vi "Main.vi"() -> ()   [LabVIEW 2013]
doc: "This template is for the Queued Message Handler design pattern.\n\nThe Event Handling Loop generates messages based on user interface actions.\n\nThe Message Handling Loop processes messages generated by the Event Handling Loop, or by other messages. The messages are string values, so new messages can be added easily to the Message Cases case structure in the Message Handling Loop. Each message cluster can also provide an optional value for Message Data, which is a variant that can be converted to whatever message-specific data is required."
uses:
  controls/UI Data.ctl
  support/Message Queue/Enqueue Message (Single).vi
  support/Message Queue/Enqueue Message (Array).vi
  <vilib>/Utility/error.llb/Error Cluster From Error Code.vi
  <vilib>/ErrorRing/Error Ring.xnode
  support/Message Queue/Message Queue.lvlib
  support/User Event - Stop/User Event - Stop.lvlib
panel:
  out "Praca":bool
  out "Display <Replace Me>":string
  in  "Do Something Else <Replace Me>":bool
  in  "Do Something <Replace Me>":bool
  in  "Exit":bool
  # "These controls have associated \"Value Changed\" events configured in the Event Structure on the diagram.\n\nReplace them (and reconfigure the Event Structure) with the controls you need for your application."
  # "This template is for the Queued Message Handler design pattern.\n\nSee the block diagram for more information on how to use this template."
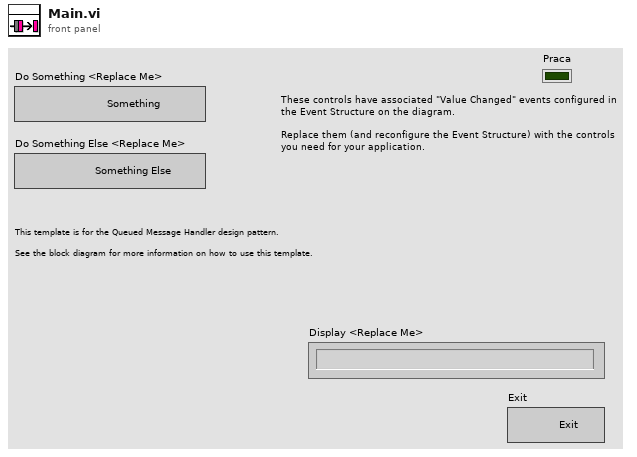
[diagram p1: front panel]
types:
  T1 = typedef "UI Data.ctl" = cluster{"Boolean <Replace Me>":bool, "String <Replace Me>":string, "Numeric <Replace Me>":dbl, "Do Something Ref":refnum<vi>, "Do Something Else Ref":refnum<vi>, "Data Display Ref":refnum<vi>, "Exit Button Ref":refnum<vi>}
  T2 = typedef "Message Queue.lvlib/All Message Queues.ctl" = cluster{"UI":refnum<queue>}
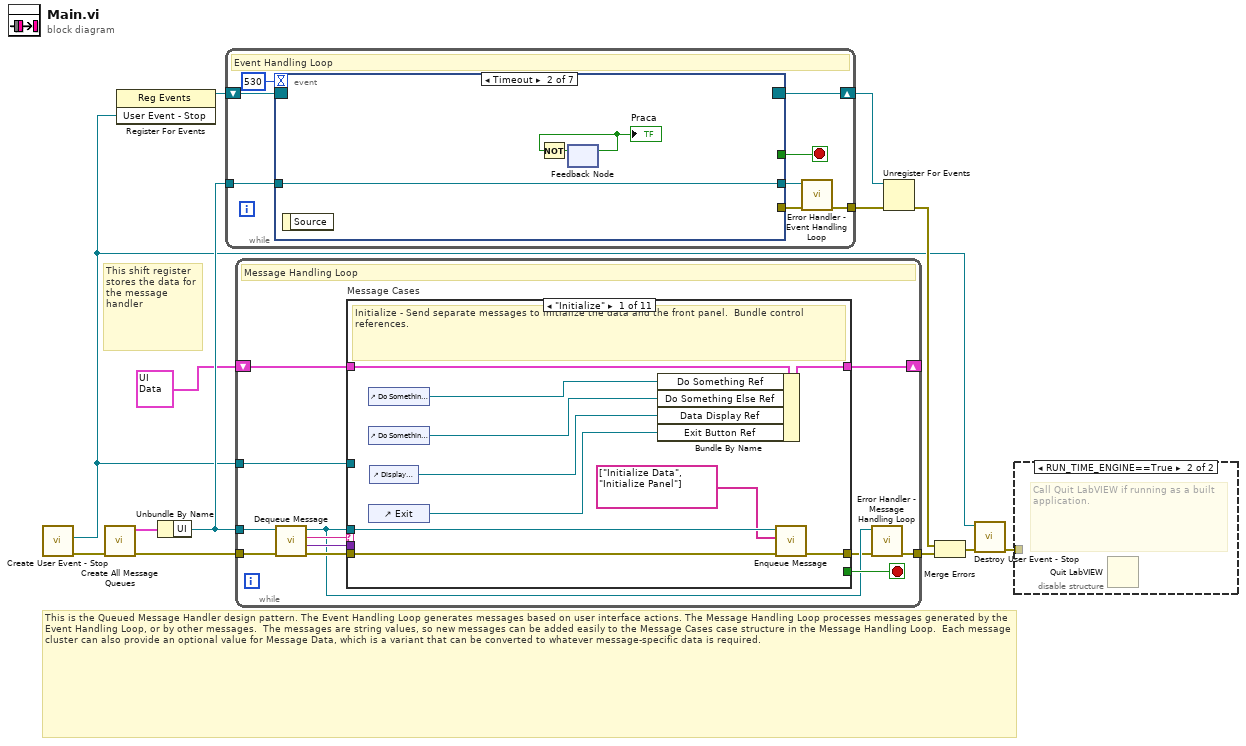
[diagram p0: block diagram]
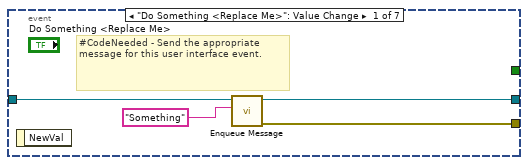
[diagram p3: hidden frame]
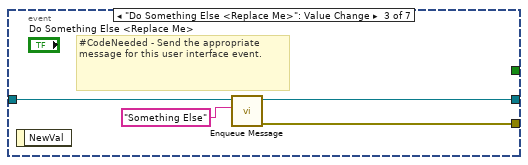
[diagram p4: hidden frame]
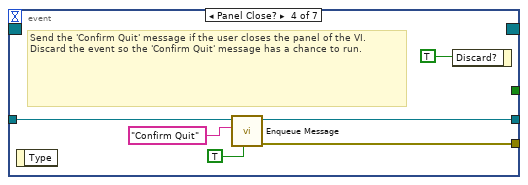
[diagram p5: hidden frame]
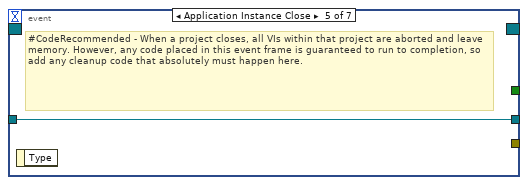
[diagram p6: hidden frame]
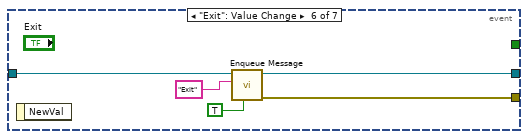
[diagram p7: hidden frame]
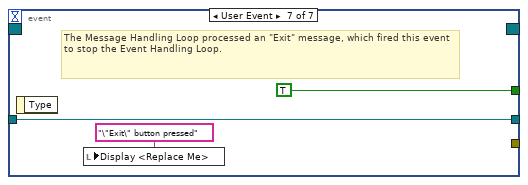
[diagram p8: hidden frame]
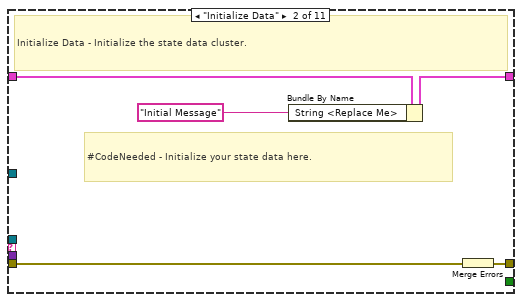
[diagram p9: hidden frame]
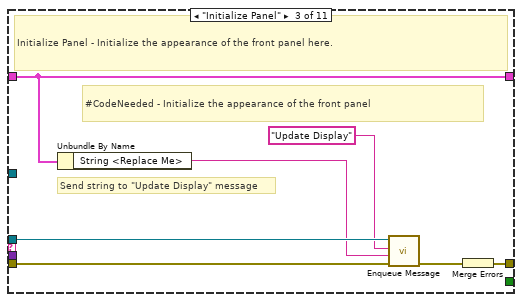
[diagram p10: hidden frame]
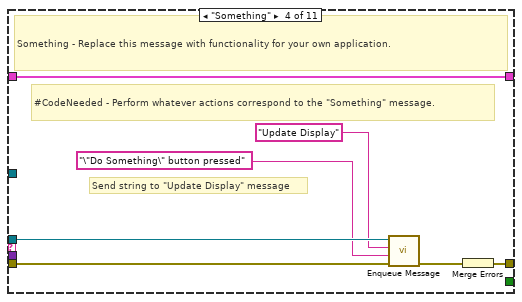
[diagram p11: hidden frame]
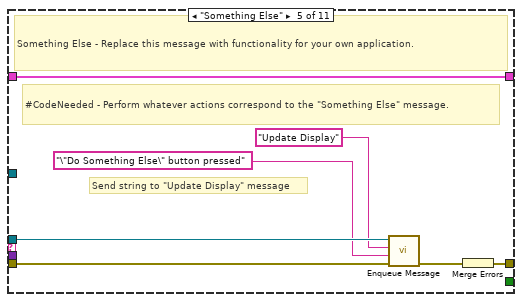
[diagram p12: hidden frame]
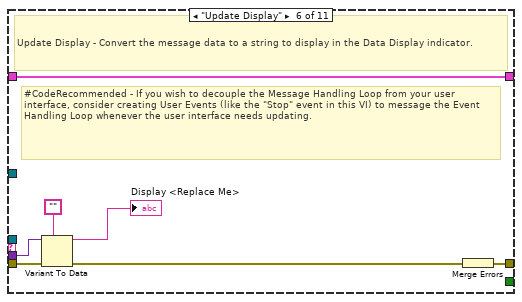
[diagram p13: hidden frame]
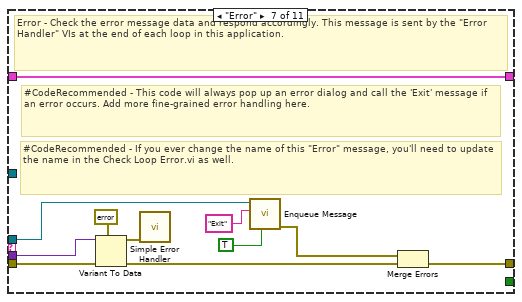
[diagram p14: hidden frame]
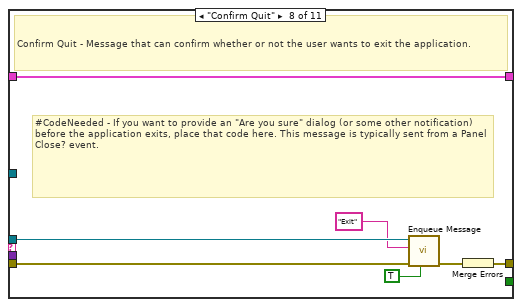
[diagram p15: hidden frame]
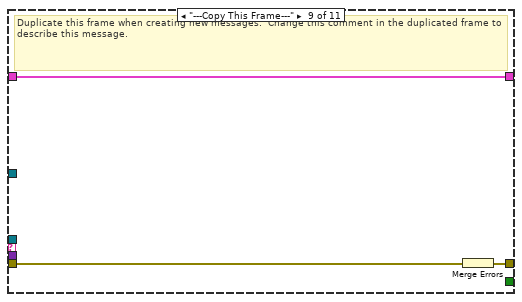
[diagram p16: hidden frame]
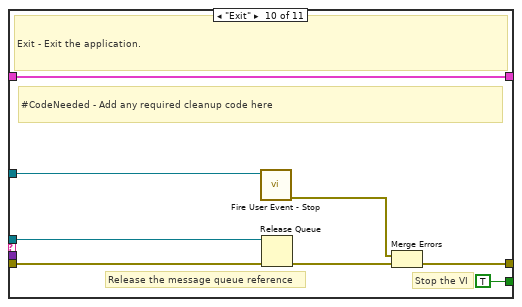
[diagram p17: hidden frame]
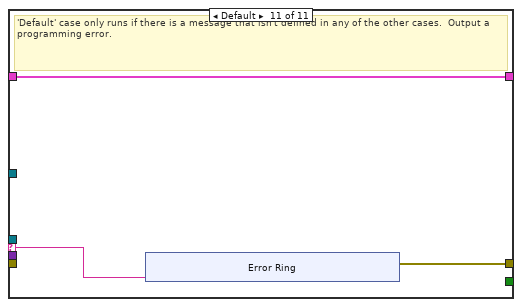
[diagram p18: hidden frame]
diagram:
  # "This is the Queued Message Handler design pattern. The Event Handling Loop generates messages based on user interface actions. The Message Handling Loop processes messages generated by the Event Handling Loop, or by other messages.  The messages are string values, so new messages can be added easily to the Message Cases case structure in the Message Handling Loop.  Each message cluster can also provide an optional value for Message Data, which is a variant that can be converted to whatever message-specific data is required."
  # "This shift register stores the data for the message handler"
  n1 = call "Create User Event - Stop.vi"() -> ("error out"=w9:errorcluster, "User Event - Stop"=w2:refnum<user-event>)  [unwired: 10 in]
  n2 = call "Create All Message Queues.vi"("error in (no error)"=w9) -> ("error out"=w13:errorcluster, "Message Queues out"=w12:T2)  [unwired: 9 in]
  n3 = register-events(w2) -> (reference out=w1:refnum<event-registration>)  [unwired: 2 in, 1 out]
  n4 = Unbundle By Name(w12) -> ("UI"=w10:refnum<queue>)
  n5 = while {
    tunnel: w10 -> [w21]
    shift-right: [w19] -> w6
    shift-left: w1 -> [w20]
    tunnel: [w15] -> w3
    stop <- w17 stop-if-true
    # "Event Handling Loop"
    n6 = event shown="[1] Timeout" {
      selector: w20 -> [_ _ _ _ _ _ _]
      dyn-events: [_ _ _ _ _ _ _] -> w19
      timeout: 530 -> [_ _ _ _ _ _ _]
      tunnel: [_ _ _ _ _ _ TRUE ("Discard?")] -> w17
      tunnel: w21 -> [w25 w28 w32 w37 w39 w44 w47]
      tunnel: [w22 _ w29 w36 _ w43 _] -> w18
      tunnel: [w24 w28 w31 w35 w39 w42 w47] -> w16
      event "Do Something <Replace Me>": Value Change {
        # "#CodeNeeded - Send the appropriate message for this user interface event."
        n7 = event-data() -> ()  [unwired: 1 in, 1 out]
        n8 = call-poly "Enqueue Message.vi"("Message"="Something", "Message Queue"=w25) -> ("error out"=w22:errorcluster, "dup Message Queue"=w24:refnum<queue>)  [unwired: 8 in]
      }
      event Timeout {
        n9 = event-data() -> ()  [unwired: 1 in, 1 out]
        n10 = feedback #1() -> (w26:bool)  [unwired: 1 in]
        "Praca" <- w26
        n11 = Not(x=w26) -> (.not. x?=w27:bool)
        n12 = feedback-in #1(w27) -> ()
      }
      event "Do Something Else <Replace Me>": Value Change {
        # "#CodeNeeded - Send the appropriate message for this user interface event."
        n13 = event-data() -> ()  [unwired: 1 in, 1 out]
        n14 = call-poly "Enqueue Message.vi"("Message"="Something Else", "Message Queue"=w32) -> ("error out"=w29:errorcluster, "dup Message Queue"=w31:refnum<queue>)  [unwired: 8 in]
      }
      event Panel Close? {
        # "Send the 'Confirm Quit' message if the user closes the panel of the VI. Discard the event so the 'Confirm Quit' message has a chance to run."
        n15 = event-data() -> ()  [unwired: 1 in, 1 out]
        n16 = call-poly "Enqueue Message.vi"("Priority Message? (F)"=TRUE, "Message"="Confirm Quit", "Message Queue"=w37) -> ("error out"=w36:errorcluster, "dup Message Queue"=w35:refnum<queue>)  [unwired: 7 in]
        n17 = event-data("Discard?"=TRUE) -> ()  [unwired: 1 in, 1 out]
      }
      event Application Instance Close {
        # "#CodeRecommended - When a project closes, all VIs within that project are aborted and leave memory. However, any code placed in this event frame is guaranteed to run to completion, so add any cleanup code that absolutely must happen here."
        n18 = event-data() -> ()  [unwired: 1 in, 1 out]
      }
      event "Exit": Value Change {
        n19 = event-data() -> ()  [unwired: 1 in, 1 out]
        n20 = call-poly "Enqueue Message.vi"("Priority Message? (F)"=TRUE, "Message"="Exit", "Message Queue"=w44) -> ("error out"=w43:errorcluster, "dup Message Queue"=w42:refnum<queue>)  [unwired: 7 in]
      }
      event User Event {
        # "The Message Handling Loop processed an \"Exit\" message, which fired this event to stop the Event Handling Loop."
        n21 = event-data() -> ()  [unwired: 1 in, 1 out]
        n22 = local write "Display <Replace Me>"("\"Exit\" button pressed" ("VI Stopped")) -> ()
      }
    }
    n23 = call "Error Handler - Event Handling Loop.vi"("error in (no error)"=w18, "Message Queue"=w16) -> ("dup error in"=w15:errorcluster)  [unwired: 8 in, 1 out]
  }
  n24 = while {
    tunnel: w10 -> [w51]
    shift-right: [w58] -> _
    shift-left: T1 {"Boolean <Replace Me>"=FALSE, "String <Replace Me>"="", "Numeric <Replace Me>"=0.0, "Do Something Ref"=refnum, "Do Something Else Ref"=refnum, "Data Display Ref"=refnum, "Exit Button Ref"=refnum} ("Data Cluster") -> [w59]
    tunnel: w2 -> [w56]
    tunnel: w13 -> [w55]
    tunnel: [w49] -> w11
    stop <- w57 stop-if-true
    # "Message Handling Loop"
    n25 = call "Dequeue Message.vi"("error in (no error)"=w55, "Message Queue"=w51) -> ("error out"=w54:errorcluster, "Message Data"=w52:variant, "Message"=w53:string, "dup Message Queue"=w50:refnum<queue>)  [unwired: 6 in]
    n26 = case "Message Cases" shown="\"Initialize\"" w53 {
      selector: w53 -> [_ _ _ _ _ _ _ _ _ _ w132]
      tunnel: w50 -> [w67 _ w78 w84 w91 _ w105 w116 _ w131 _]
      tunnel: w54 -> [w68 w74 w79 w86 w93 w100 w113 w120 w123 w126 _]
      tunnel: [w69 w70 w80 w87 w94 w101 w106 w118 w121 w127 w133] -> w48
      tunnel: w59 -> [w66 w73 w81 w88 w95 w102 w112 w119 w122 w130 w134]
      tunnel: [w65 w72 w81 w88 w95 w102 w112 w119 w122 w130 w134] -> w58
      tunnel: [_ _ _ _ _ _ _ _ _ TRUE _] -> w57
      tunnel: w52 -> [_ _ _ _ _ w99 w111 _ _ _ _]
      tunnel: w56 -> [_ _ _ _ _ _ _ _ _ w125 _]
      frame "Initialize" {
        # "Initialize - Send separate messages to initialize the data and the front panel.  Bundle control references."
        n27 = control-ref of="Do Something <Replace Me>"() -> (w64:refnum<vi>)
        n28 = control-ref of="Do Something Else <Replace Me>"() -> (w63:refnum<vi>)
        n29 = control-ref of="Exit"() -> (w61:refnum<vi>)
        n30 = control-ref of="Display <Replace Me>"() -> (w62:refnum<vi>)
        n31 = Bundle By Name(cluster=w66, "Do Something Ref"=w64, "Do Something Else Ref"=w63, "Data Display Ref"=w62, "Exit Button Ref"=w61) -> (w65:T1)
        n32 = call-poly "Enqueue Message.vi"("error in (no error)"=w68, "Message Array"=string[] ["Initialize Data", "Initialize Panel"], "Message Queue"=w67) -> ("error out"=w69:errorcluster)  [unwired: 7 in, 1 out]
      }
      frame "Initialize Data" {
        # "#CodeNeeded - Initialize your state data here."
        # "Initialize Data - Initialize the state data cluster."
        n33 = Bundle By Name(cluster=w73, "String <Replace Me>"="Initial Message" ("Initial Message")) -> (w72:T1)
        n34 = Merge Errors(w74) -> (w70:errorcluster)
      }
      frame "Initialize Panel" {
        # "Send string to \"Update Display\" message"
        # "#CodeNeeded - Initialize the appearance of the front panel"
        # "Initialize Panel - Initialize the appearance of the front panel here."
        n35 = Unbundle By Name(w81) -> ("String <Replace Me>"=w75:string)
        n36 = call-poly "Enqueue Message.vi"("error in (no error)"=w79, "Message Data"=w75, "Message"="Update Display", "Message Queue"=w78) -> ("error out"=w77:errorcluster)  [unwired: 6 in, 1 out]
        n37 = Merge Errors(w77) -> (w80:errorcluster)
      }
      frame "Something" {
        # "Send string to \"Update Display\" message"
        # "#CodeNeeded - Perform whatever actions correspond to the \"Something\" message."
        # "Something - Replace this message with functionality for your own application."
        n38 = call-poly "Enqueue Message.vi"("error in (no error)"=w86, "Message Data"="\"Do Something\" button pressed" ("\"Do Something\" button pressed"), "Message"="Update Display", "Message Queue"=w84) -> ("error out"=w85:errorcluster)  [unwired: 6 in, 1 out]
        n39 = Merge Errors(w85) -> (w87:errorcluster)
      }
      frame "Something Else" {
        # "Send string to \"Update Display\" message"
        # "#CodeNeeded - Perform whatever actions correspond to the \"Something Else\" message."
        # "Something Else - Replace this message with functionality for your own application."
        n40 = call-poly "Enqueue Message.vi"("error in (no error)"=w93, "Message Data"="\"Do Something Else\" button pressed" ("\"Do Something Else\" button pressed"), "Message"="Update Display", "Message Queue"=w91) -> ("error out"=w92:errorcluster)  [unwired: 6 in, 1 out]
        n41 = Merge Errors(w92) -> (w94:errorcluster)
      }
      frame "Update Display" {
        # "#CodeRecommended - If you wish to decouple the Message Handling Loop from your user interface, consider creating User Events (like the \"Stop\" event in this VI) to message the Event Handling Loop whenever the user interface needs updating."
        # "Update Display - Convert the message data to a string to display in the Data Display indicator."
        n42 = Variant To Data(error in=w100, type="", Variant=w99) -> (data=→"Display <Replace Me>":string, error out=w97:errorcluster)
        n43 = Merge Errors(w97) -> (w101:errorcluster)
      }
      frame "Error" {
        # "#CodeRecommended - If you ever change the name of this \"Error\" message, you'll need to update the name in the Check Loop Error.vi as well."
        # "#CodeRecommended - This code will always pop up an error dialog and call the 'Exit' message if an error occurs. Add more fine-grained error handling here."
        # "Error - Check the error message data and respond accordingly. This message is sent by the \"Error Handler\" VIs at the end of each loop in this application."
        n44 = Variant To Data(error in=w113, type=errorcluster {"status"=FALSE, "code"=0, "source"=""} ("error constant"), Variant=w111) -> (data=w109:errorcluster, error out=w108:errorcluster)
        n45 = call <vilib>:"Simple Error Handler.vi"("error in (no error)"=w109) -> ()  [unwired: 4 in, 5 out]
        n46 = call-poly "Enqueue Message.vi"("Priority Message? (F)"=TRUE, "Message"="Exit", "Message Queue"=w105) -> ("error out"=w107:errorcluster)  [unwired: 7 in, 1 out]
        n47 = Merge Errors(w107, w108) -> (w106:errorcluster)
      }
      frame "Confirm Quit" {
        # "#CodeNeeded - If you want to provide an \"Are you sure\" dialog (or some other notification) before the application exits, place that code here. This message is typically sent from a Panel Close? event."
        # "Confirm Quit - Message that can confirm whether or not the user wants to exit the application."
        n48 = call-poly "Enqueue Message.vi"("Priority Message? (F)"=TRUE, "error in (no error)"=w120, "Message"="Exit", "Message Queue"=w116) -> ("error out"=w117:errorcluster)  [unwired: 6 in, 1 out]
        n49 = Merge Errors(w117) -> (w118:errorcluster)
      }
      frame "---Copy This Frame---" {
        # "Duplicate this frame when creating new messages.  Change this comment in the duplicated frame to describe this message."
        n50 = Merge Errors(w123) -> (w121:errorcluster)
      }
      frame "Exit" {
        # "Stop the VI"
        # "Release the message queue reference"
        # "#CodeNeeded - Add any required cleanup code here"
        # "Exit - Exit the application."
        n51 = call "Fire User Event - Stop.vi"("User Event - Stop"=w125) -> ("error out"=w124:errorcluster)  [unwired: 10 in]
        n52 = Release Queue(queue=w131, error in (no error)=w126) -> (error out=w128:errorcluster)  [unwired: 1 in, 2 out]
        n53 = Merge Errors(w124, w128) -> (w127:errorcluster)
      }
      frame Default {
        # "'Default' case only runs if there is a message that isn't defined in any of the other cases.  Output a programming error."
        n54 = xnode "Error Ring"("parameter 0"=w132) -> ("error out"=w133:errorcluster)
      }
    }
    n55 = call "Error Handler - Message Handling Loop.vi"("error in (no error)"=w48, "Message Queue"=w50) -> ("dup error in"=w49:errorcluster)  [unwired: 8 in, 1 out]
  }
  n56 = Unregister For Events(event registration refnum=w6, error in=w3) -> (error out=w7:errorcluster)
  n57 = Merge Errors(w7, w11) -> (w8:errorcluster)
  n58 = call "Destroy User Event - Stop.vi"("error in (no error)"=w8, "User Event - Stop"=w2) -> ("error out"=w4:errorcluster)  [unwired: 9 in]
  n59 = disable-structure shown="RUN_TIME_ENGINE==True" {
    disable-tunnel: w4 -> [_ _]
    frame condition #0 (active) {
    }
    frame condition #1 {
      # "Call Quit LabVIEW if running as a built application."
      n60 = Quit LabVIEW() -> ()  [unwired: 1 in]
    }
  }
